vi "event_log_engine.vi"() -> (0 "error out":errorcluster, 3 "element":T1)   [LabVIEW 2017, in "labview-standard-library.lvlib"]
uses:
  labview-standard-library.lvlib
  Time&Event_cluster.ctl
  Event_logging_state_control.ctl
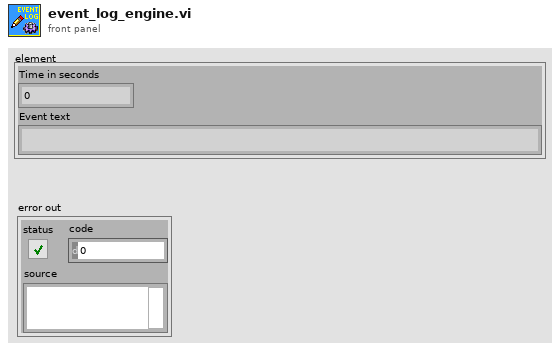
[diagram p1: front panel]
types:
  T1 = typedef "labview-standard-library.lvlib/Time&Event_cluster.ctl" = cluster{"Time in seconds":dbl, "Event text":string}
  T2 = typedef "labview-standard-library.lvlib/Event_logging_state_control.ctl" = enum16{"Write", "Publish to txt", "Publish to csv"}
  T3 = enum16{"open", "replace", "create", "open or create", "replace or create", "replace or create with confirmation"}
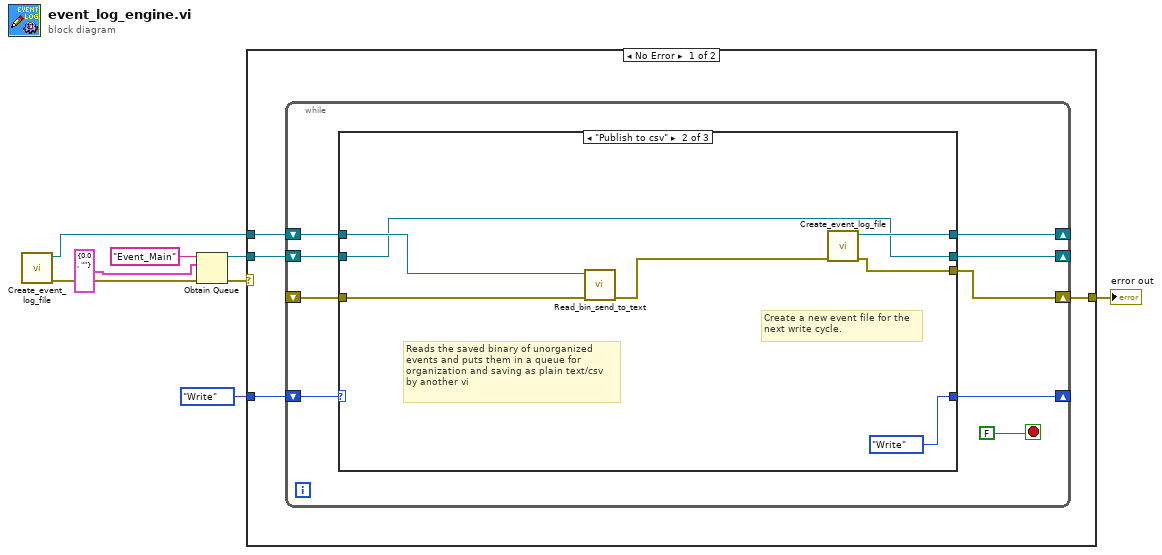
[diagram p0: block diagram]
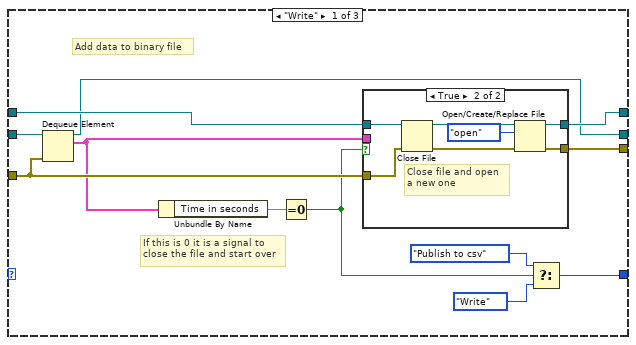
[diagram p2: hidden frame]
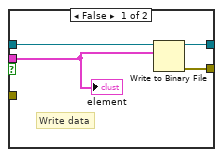
[diagram p3: hidden frame]
diagram:
  n1 = call "Create_event_log_file.vi"() -> ("error out"=w5:errorcluster, "Log file refnum out"=w6:refnum<file>)  [unwired: 9 in, 1 out]
  n2 = Obtain Queue(name (unnamed)="Event_Main", element data type=T1 {"Time in seconds"=0.0, "Event text"=""} ("Cluster"), error in (no error)=w5) -> (queue out=w3:refnum<queue>, error out=w4:errorcluster)  [unwired: 2 in, 1 out]
  n3 = case shown="No Error" w4 {
    selector: w4 -> [_ w56]
    tunnel: w3 -> [w12 _]
    tunnel: w6 -> [w11 _]
    tunnel: Event_logging_state_control."Write" -> [w10 _]
    tunnel: [w9 w56] -> w1
    frame No Error {
      n4 = while {
        shift-right: [w21] -> _
        shift-left: w11 -> [w19]
        shift-right: [w20] -> w9
        shift-left: _ -> [w17]
        shift-right: [w13] -> _
        shift-left: w12 -> [w15]
        shift-right: [w14] -> _
        shift-left: w10 -> [w16]
        stop <- FALSE stop-if-true
        n5 = case shown="\"Publish to csv\"" w16 {
          selector: w16 -> [_ _ w52]
          tunnel: [w33 w48 w55] -> w21
          tunnel: [w32 w47 w53] -> w20
          tunnel: w19 -> [w31 w51 w55]
          tunnel: w17 -> [w26 w50 w53]
          tunnel: w15 -> [w30 w45 w54]
          tunnel: [w29 Event_logging_state_control."Write" w52] -> w14
          tunnel: [w22 w45 w54] -> w13
          frame "Write" {
            # "If this is 0 it is a signal to\nclose the file and start over"
            # "Add data to binary file"
            n6 = Dequeue Element(queue=w30, error in (no error)=w26) -> (queue out=w22:refnum<queue>, element=w25:T1)  [unwired: 1 in, 2 out]
            n7 = Unbundle By Name(w25) -> ("Time in seconds"=w24:dbl)
            n8 = Equal To 0?(x=w24) -> (x = 0?=w23:bool)
            n9 = case shown="True" w23 {
              tunnel: [w37 w43] -> w33
              tunnel: [w36 w44] -> w32
              tunnel: w31 -> [w35 w41]
              tunnel: w25 -> [w34 _]
              tunnel: w26 -> [_ w40]
              frame False {
                # "Write data"
                n10 = Write to Binary File(file (use dialog)=w35, data=w34) -> (refnum out=w37:refnum<file>, error out=w36:errorcluster)  [unwired: 4 in, 1 out]
                "element" <- w34
              }
              frame True {
                # "Close file and open\na new one"
                n11 = Close File(refnum=w41, error in=w40) -> (path=w38:path, error out=w39:errorcluster)
                n12 = Open/Create/Replace File(file path (use dialog)=w38, error in=w39, operation (0:open)=T3."open") -> (refnum out=w43:refnum<file>, error out=w44:errorcluster)  [unwired: 3 in, 1 out]
              }
            }
            n13 = Select(t=Event_logging_state_control."Publish to csv", s=w23, f=Event_logging_state_control."Write") -> (s? t:f=w29:T2)
          }
          frame "Publish to csv" {
            # "Create a new event file for the\nnext write cycle."
            # "Reads the saved binary of unorganized\nevents and puts them in a queue for \norganization and saving as plain text/csv\nby another vi"
            n14 = call "Read_bin_send_to_text.vi"("error in (no error)"=w50, "Byte Stream File in"=w51) -> ("error out"=w46:errorcluster)  [unwired: 9 in]
            n15 = call "Create_event_log_file.vi"("error in"=w46) -> ("error out"=w47:errorcluster, "Log file refnum out"=w48:refnum<file>)  [unwired: 8 in, 1 out]
          }
          frame "Publish to txt" {
            # "Unused (Publish to CSV does the same thing)"
          }
        }
      }
    }
    frame Error {
    }
  }
  "error out" <- w1
